vi "parseOdometry.vi"(0 "msg in":string) -> (4 "Odometry":T1, 5 "msg out":string, 6 "Header":T2, 7 "child_frame_id":string, 8 "Pose 2D":cluster{"x":dbl, "y":dbl})   [LabVIEW 2014]
doc: "Parses a message into an odometry"
uses:
  <vilib>/Tufts CEEO ROS for LabVIEW Software/ROS/MessageParsing/std_msgs/subs/parse_string_scalar.vi
  <vilib>/Tufts CEEO ROS for LabVIEW Software/ROS/MessageParsing/std_msgs/subs/parse_float64_scalar.vi
panel:
  out "error out 2":errorcluster
  out "error out":errorcluster
  in  "error in":errorcluster
  out "msg out 2":string
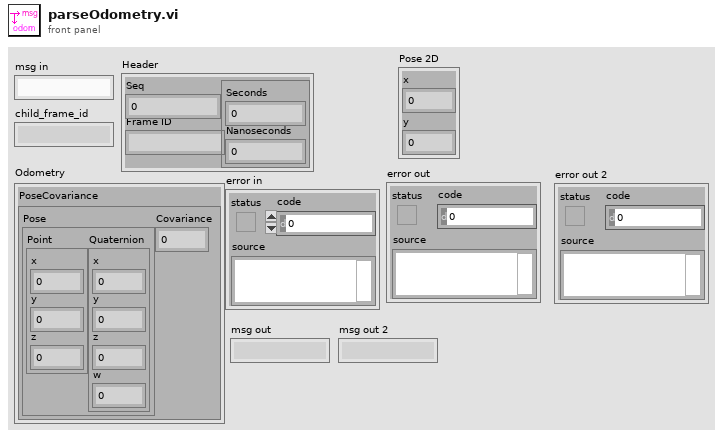
[diagram p1: front panel]
types:
  T1 = cluster{"PoseCovariance":cluster{"Pose":cluster{"Point":cluster{"x":dbl, "y":dbl, "z":dbl}, "Quaternion":cluster{"x":dbl, "y":dbl, "z":dbl, "w":dbl}}, "Covariance":dbl}}
  T2 = cluster{"Seq":u32, "Frame ID":string, "Timestamp":cluster{"Seconds":i32, "Nanoseconds":i32}}
  T3 = cluster{"Pose":cluster{"Point":cluster{"x":dbl, "y":dbl, "z":dbl}, "Quaternion":cluster{"x":dbl, "y":dbl, "z":dbl, "w":dbl}}, "Covariance":dbl}
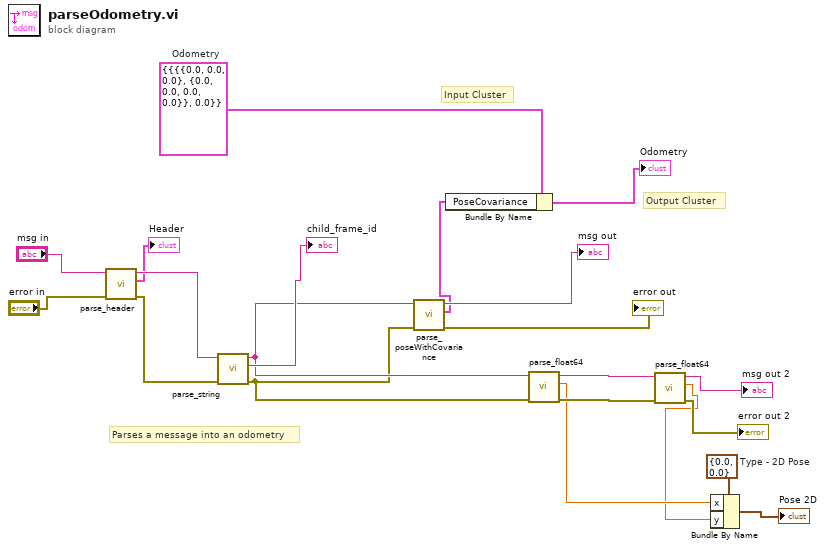
[diagram p0: block diagram]
diagram:
  w4 = cluster{"x":dbl, "y":dbl} {"x"=0.0, "y"=0.0}  # Type - 2D Pose
  w17 = T1 {"PoseCovariance"={"Pose"={"Point"={"x"=0.0, "y"=0.0, "z"=0.0}, "Quaternion"={"x"=0.0, "y"=0.0, "z"=0.0, "w"=0.0}}, "Covariance"=0.0}}  # Odometry
  # "Input Cluster"
  # "Output Cluster"
  # "Parses a message into an odometry"
  n1 = call <vilib>:"parse_header.vi"("error in"="error in", "msg in"="msg in") -> ("error out"=w8:errorcluster, "Header"=→"Header":T2, "msg out"=w20:string)  [unwired: 3 in]
  n2 = call-poly <vilib>:"parse_string.vi"("error in"=w8, "msg in"=w20) -> ("error out"=w7:errorcluster, "string"=→"child_frame_id":string, "msg out"=w10:string)  [unwired: 3 in]
  n3 = call <vilib>:"parse_poseWithCovariance.vi"("error in (no error)"=w7, "msg in"=w10) -> ("error out"=→"error out":errorcluster, "PoseCovariance"=w14:T3, "msg out"=→"msg out":string)  [unwired: 3 in]
  n4 = Bundle By Name "Bundle By Name"(cluster=w17, "PoseCovariance"=w14) -> (→"Odometry":T1)
  n5 = call-poly <vilib>:"parse_float64.vi"("error in"=w7, "msg in"=w10) -> ("error out"=w12:errorcluster, "number"=w3:dbl, "msg out"=w13:string)  [unwired: 3 in]
  n6 = call-poly <vilib>:"parse_float64.vi"("error in"=w12, "msg in"=w13) -> ("error out"=→"error out 2":errorcluster, "number"=w2:dbl, "msg out"=→"msg out 2":string)  [unwired: 3 in]
  n7 = Bundle By Name(cluster=w4, "x"=w3, "y"=w2) -> (→"Pose 2D":cluster{"x":dbl, "y":dbl})
